vi "WPI_CameraStart Asynchronous VI.vi"(7 "Control Name":string, 8 "error in (no error)":errorcluster, 9 "Auto Dispose Reference":bool, 10 "VI Refnum":refnum<vi>, 11 "Value":variant) -> (0 "error out":errorcluster, 2 "VI Refnum Dup":refnum<vi>)   [LabVIEW 2017]
doc: "This software is licensed. Open the labview\\readme\\WPI Robotics Library Open Source License.txt file for more information."
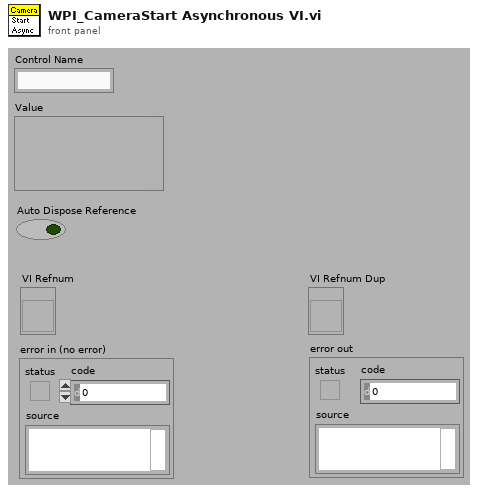
[diagram p1: front panel]
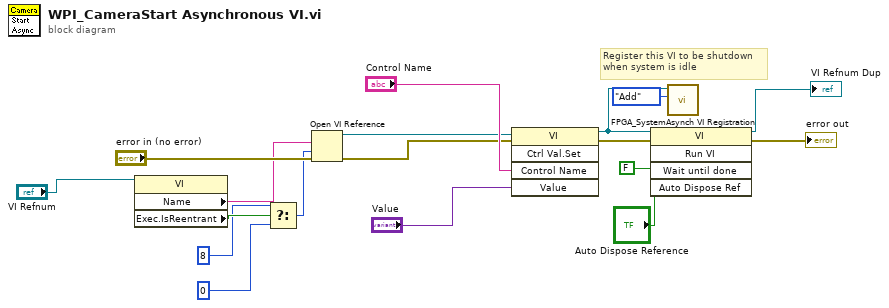
[diagram p0: block diagram]
diagram:
  # "Register this VI to be shutdown\nwhen system is idle"
  n1 = property class="VI"(reference="VI Refnum") -> ("Name"=w9:string, "Exec.IsReentrant"=w7:bool)  [unwired: 1 in, 2 out]
  n2 = Select(t=8, s=w7, f=0) -> (s? t:f=w4:i32)
  n3 = Open VI Reference(vi path=w9, options=w4, error in (no error)="error in (no error)") -> (vi reference=w10:refnum<vi>, error out=w11:errorcluster)  [unwired: 1 in, 2 out]
  n4 = invoke class="VI" method="Ctrl Val.Set"(reference=w10, error in=w11, "Control Name"="Control Name", "Value"="Value") -> (reference out=w2:refnum<vi>, error out=w12:errorcluster)  [unwired: 1 in, 3 out]
  n5 = invoke class="VI" method="Run VI"(reference=w2, error in=w12, "Wait until done"=FALSE ("Wait Until Done"), "Auto Dispose Ref"="Auto Dispose Reference") -> (reference out=→"VI Refnum Dup":refnum<vi>, error out=→"error out":errorcluster)  [unwired: 1 in, 3 out]
  n6 = call <vilib>:"FPGA_SystemAsynch VI Registration.vi"("Operation"=enum16{"Get", "Add", "Remove"}."Add", "VI Refnum"=w2) -> ()  [unwired: 10 out]
